vi "TreeInfor.vi"() -> (2 "Array":string[][](array[string])=[["Device", "Device", "0", "List.png"], ["PXI-6251", "PXI6251", "1", "Card.png"], ["Analog input", "ai", "2", "Channel.png"], ["PXI-6120", "PXI6120", "1", "Card.png"], ["Analog input", "Sai", "2", "DRP.png"], ["PXI-6704", "PXI6704", "1", "Card.png"], ["Analog output", "ao", "2", "Channel.png"], ["PXI-6514", "PXI651", "1", "Card.png"], ["Digital I/O", "dio", "2", "Channel.png"], ["PXI-8341", "PXI8341", "1", "Card.png"], ["RS 485", "com", "2", "Channel.png"]])   [LabVIEW 2017]
panel:
  in  "Tree":string[][](table)=[["Device", "Device", "0", "List.png"], ["PXI-6251", "PXI6251", "1", "Card.png"], ["Analog input", "ai", "2", "Channel.png"], ["PXI-6704", "PXI6704", "1", "Card.png"], ["Analog output", "ao", "2", "Channel.png"], ["PXI-6515", "PXI6514", "1", "Card.png"], ["Digital I/O", "dio", "2", "Channel.png"], ["PXI-8431_6slot", "PXI8431_6", "1", "Card.png"], ["RS 485", "com_slot6", "2", "Channel.png"], ["PXI-6602", "PXI6602", "1", "Card.png"], ["Time I/O", "tio", "2", "Channel.png"]]
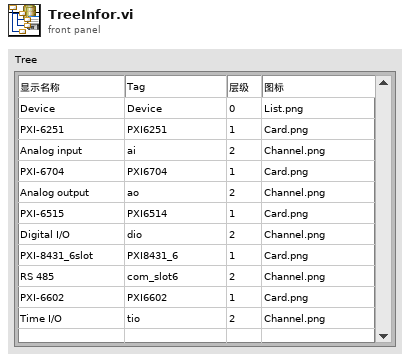
[diagram p1: front panel]
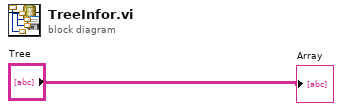
[diagram p0: block diagram]
diagram:
  "Array" <- "Tree"
